vi "G heatmap=f(orbital angle, E_mol)_on Au.vi"() -> ()   [LabVIEW 2016]
uses:
  <vilib>/Math Plots/3D Math Plots/3D Contour/3D Contour XCtrl/3D Contour.xctl
  <vilib>/Math Plots/3D Math Plots/3D Contour/3D Contour Datatype/3D Contour Datatype.lvclass
  <vilib>/Analysis/1siggen.llb/Ramp Pattern by Samples.vi
  <vilib>/Math Plots/3D Math Plots/3D Contour/3D Contour Datatype/Public/Plot Helper (Vector).vi
  <vilib>/Utility/file.llb/Write Delimited Spreadsheet (DBL).vi
  <vilib>/Analysis/NI_AALBase.lvlib
  <vilib>/Math Plots/3D Math Plots/3D Plot/3D Plot Datatype/3D Plot Datatype.lvclass
  <vilib>/Analysis/NI_AALPro.lvlib
panel:
  out "SDOS(angle, e_iso) for t(d-head)_sum dz2 & dyz 2":refnum<class "3D Plot Datatype.lvclass">[](xcontrol)
  out "unweighted pz SDOS \n@ intercept":dbl
  out "t^2_pz-mol":dbl
  out "t_pz-mol":dbl
  in  "eta (pp sigma)":i32=2
  in  "t_pz band":dbl=4.15 format="%.2f"
  in  "e_pz band (vs. E_F)":dbl=8.19 format="%.2f"
  out "pz SDOS top (/eV/atom)":dbl=0.118 format="%.3f"
  in  "turn on dyz":bool=TRUE
  in  "turn on dz2":bool=TRUE
  out "<= min[dnn]?":bool
  out "e_FMO after dz2\n(vs. E_F) <=>\nintercept on E\ndz2 band-mol":dbl
  out "e_FMO after sp \n(vs. E_F) <=>\nintercept on E\nsp band-mol":dbl
  out "intercept on E\ndyz band-mol":dbl
  out "graphical sol_dyz band-mol":cluster{"Ramp Pattern":dbl[], dbl[]}[](graph)
  out "delta shift by d band \n(w.r.t. e_FMO coupled to s/p then dz2 )":dbl
  out "unweighted dyz SDOS \n@intercept":dbl
  in  "e_dyz band \n(vs. E_F)":dbl=-3.41 format="%.2f"
  in  "t_dyz band":dbl=1.1 format="%.2f"
  out "dyz SDOS top \n(/eV/atom)":dbl=0.793 format="%.3f"
  out "log(G/G0)=f(angle, e_iso) for t(sp-head)":refnum<class "3D Plot Datatype.lvclass">[](xcontrol)
  in  "min dnn (A)\nby induction":dbl=2.1 format="%.3g"
  out "peak value":dbl
  out "unweighted pxy SDOS \n@ intercept":dbl
  out "t^2_pxy-mol":dbl
  out "pxy SDOS top (/eV/atom)":dbl=0.118 format="%.3f"
  in  "e_pxy band (vs. E_F)":dbl=11.01 format="%.2f"
  in  "t_pxy band":dbl=6.11 format="%.2f"
  out "angle > ini?":bool
  in  "dnn shrinking \nrate\n(A/increment)":dbl=0.0094 format="%.4g"
  in  "induction rate\n(_-fold of increment)":dbl=1.9850000000000005 format="%.3g"
  in  "orbital angle \nstarting induction":dbl=46.809999999999995 format="%.2g"
  out "unweighted dz2 SDOS \n@intercept":dbl
  out "unweighted s SDOS \n@ intercept":dbl
  out "dz2 SDOS top \n(/eV/atom)":dbl=0.793 format="%.3f"
  out "s SDOS top (/eV/atom)":dbl=0.118 format="%.3f"
  in  "eta scaling for sp":dbl=0.417 format="%.3f"
  in  "name (d band)":string="on Au 5dz2 5dyz"
  in  "saving path_heatmap (d band)":path=path "C:/Users/NTU/Desktop/project_BiUPD & PbUPD/modelling/general heatmap all head_on Au"
  in  "save heatmap \n(d band)?":bool
  out "final ELA(angle, e_iso  for t(sp-head))":refnum<class "3D Plot Datatype.lvclass">[](xcontrol)
  out "delta(angle, e_iso) for t(d-head)_sum dz2 & dyz":refnum<class "3D Plot Datatype.lvclass">[](xcontrol)
  out "delta(angle, e_iso) for t(sp-head)_only s":refnum<class "3D Plot Datatype.lvclass">[](xcontrol)
  out "delta shift by dz2 band \n(w.r.t. e_FMO coupled to s/p )":dbl
  out "delta shift by sp band":dbl
  in  "dnn (pi) dyz":dbl=2.57 format="%0.2f"
  out "Gamma(angle, e_iso) for t(sp-head)_sum s pz py":refnum<class "3D Plot Datatype.lvclass">[](xcontrol)
  out "e_FMO \n(vs. E_F)":dbl
  out "log(G/G0) matrix":dbl[][](array[numeric])
  in  "tilt (mol axis - Z axis)":dbl format="%0.2f"
  out "final ELA(angle, e_iso)  for t(d-head)":refnum<class "3D Plot Datatype.lvclass">[](xcontrol)
  out "Gamma(angle, e_iso) for t(d-head)_sum dz2 & dyz":refnum<class "3D Plot Datatype.lvclass">[](xcontrol)
  out "log(G/G0)=f(angle, e_iso) for t(d-head)":refnum<class "3D Plot Datatype.lvclass">[](xcontrol)
  out "e_FMO (y)":dbl[](array[numeric])
  out "angle\narray\nfor sigma":dbl[](array[numeric])
  in  "create heatmap":bool=TRUE
  in  "name (sp band)":string="on Au 6s 6pxy"
  in  "save heatmap \n(sp band)?":bool
  in  "saving path_heatmap (sp band)":path=path "C:/Users/NTU/Desktop/project_BiUPD & PbUPD/modelling/general heatmap all head_on Au"
  in  "lower angle":dbl=-90.0 format="%_3g"
  in  "upper angle":dbl=90.0 format="%_3g"
  in  "angle increment":dbl=0.5 format="%_3g"
  in  "lower e_iso FMO":dbl=-3.0 format="%_3g"
  in  "upper e_iso FMO":dbl=3.0 format="%_3g"
  in  "increment_iso FMO":dbl=0.03 format="%_3g"
  out "t^2_dz2-mol":dbl
  out "FWHM (eV)":dbl
  in  "dnn (pi)":dbl=2.57 format="%0.2f"
  in  "WF (eV) vs. Fermi":dbl format="%.2f"
  out "t^2_p-mol":dbl
  out "t_pxy-mol":dbl
  in  "eta (pp pi)":i32=3
  in  "start (eV)":dbl=-20.0 format="%.2f"
  in  "dnn (sigma)":dbl=2.57 format="%0.2f"
  in  "eta (sp sigma)":i32=1
  out "t_s-mol":dbl
  out "intercept on E\nsp band-mol":dbl
  out "graphical sol_sp band-mol":cluster{"Ramp Pattern":dbl[], dbl[]}[](graph)
  in  "e_s band (vs. E_F)":dbl=-0.04 format="%.2f"
  in  "t_s band":dbl=5.03 format="%.2f"
  out "E":dbl[](array[numeric])
  out "t^2_dyz-mol":dbl
  out "final ELA (eV), via \n(1) sp intercept\n(2) dz2 intercept\n(3) dyz intercept":dbl
  in  "ELD AO (pi w/ FMO) - Z axis":dbl format="%0.2f"
  out "graphical sol_dz2 band-mol":cluster{"Ramp Pattern":dbl[], dbl[]}[](graph)
  out "intercept on E\ndz2 band-mol":dbl
  out "t_dz2-mol":dbl
  out "t_dyz-mol":dbl
  in  "e_dz2 band \n(vs. E_F)":dbl=-3.8000000000000003 format="%.2f"
  in  "t_dz2 band":dbl=1.26 format="%.2f"
  in  "eta (pi)":i32=2
  in  "ELD AO (sigma w/ FMO) - Z axis":dbl format="%0.2f"
  in  "mol backbone (# n)":dbl=8.0 format="%.2f"
  in  "beta (per n)":dbl=1.0 format="%.2f"
  out "conductance G0 \n(on E_F, low bias)":dbl format="%#.3e"
  in  "eta (sigma)":i32=1
  out "transmission T(E)":cluster{"Ramp Pattern":dbl[], dbl[]}(graph)
  in  "d state R (Ang)":dbl=1.0099999999999998 format="%0.2f"
  in  "FMO - mol axis":dbl format="%0.2f"
  in  "dnn (sigma) dz2":dbl=2.57 format="%0.2f"
  in  "samples":i32=10000
  in  "end (eV)":dbl=20.0 format="%_3g"
  # "for eld-head hopping integral: \nHarrsion and S-K"
  # "for ELA & Gamma: Hilbert & Newns-Anderson-Grimley graphical method"
  # "for T(E) and G(E_F)\nLandauer formula"
  # "logG heatmap = f(t(number basis), e_iso FMO)"
  # "step2. dz2 band-mol \ncoupling"
  # "step1. s/p band-mol coupling"
  # "step3. dyz band-mol coupling"
  # "Harrison LCAO hopping integral (V)"
  # "exp decay for backbone"
  # "internuclear \nspacing, dnn (Ang)"
  # "off-diagonal element type"
  # "Au s\nc: -0.04\nt: 5.03"
  # "1 sp_sigma\n2 pp_sigma"
  # "FMO-s/p eld AO"
  # "1 sp_sigma\n2 pp_sigma"
  # "Au pz\nc: 8.19\nt: 4.15"
  # "1 sp_pi =0\n2 pp_sigma\n3 pp_pi"
  # "FMO-d eld AO"
  # "Au py\nc: 11.01\nt: 6.11"
  # "1 pd_sigma\n2 pd_pi"
  # "Au dz2\nc: -3.80\nt: 1.26"
  # "Au dyz\nc: -3.41\nt: 1.10"
  # "the avg of the two \nshould be e_ELD (vs. E_F)"
  # "1 pd_sigma\n2 pd_pi"
  # "to switch off certain interactions => set very large d (Ang)"
  # "for heatmap"
  # "for inducting effect"
  # "e_iso FMO\n (vs. E_F)"
  # "angle basis"
  # "induction"
  # "dnn"
  # "note: this is\nnot simply \nthe Gamma"
  # "to switch off certain effects => set 1 or 0"
  # "Slater-Koster t =f(bond angle)"
  # "+"
  # "一"
  # "FMO - ELD AO \nangle (sigma)"
  # "="
  # "FMO - ELD AO\n angle (pi)"
  # "="
  # "inverse \ncolor scale"
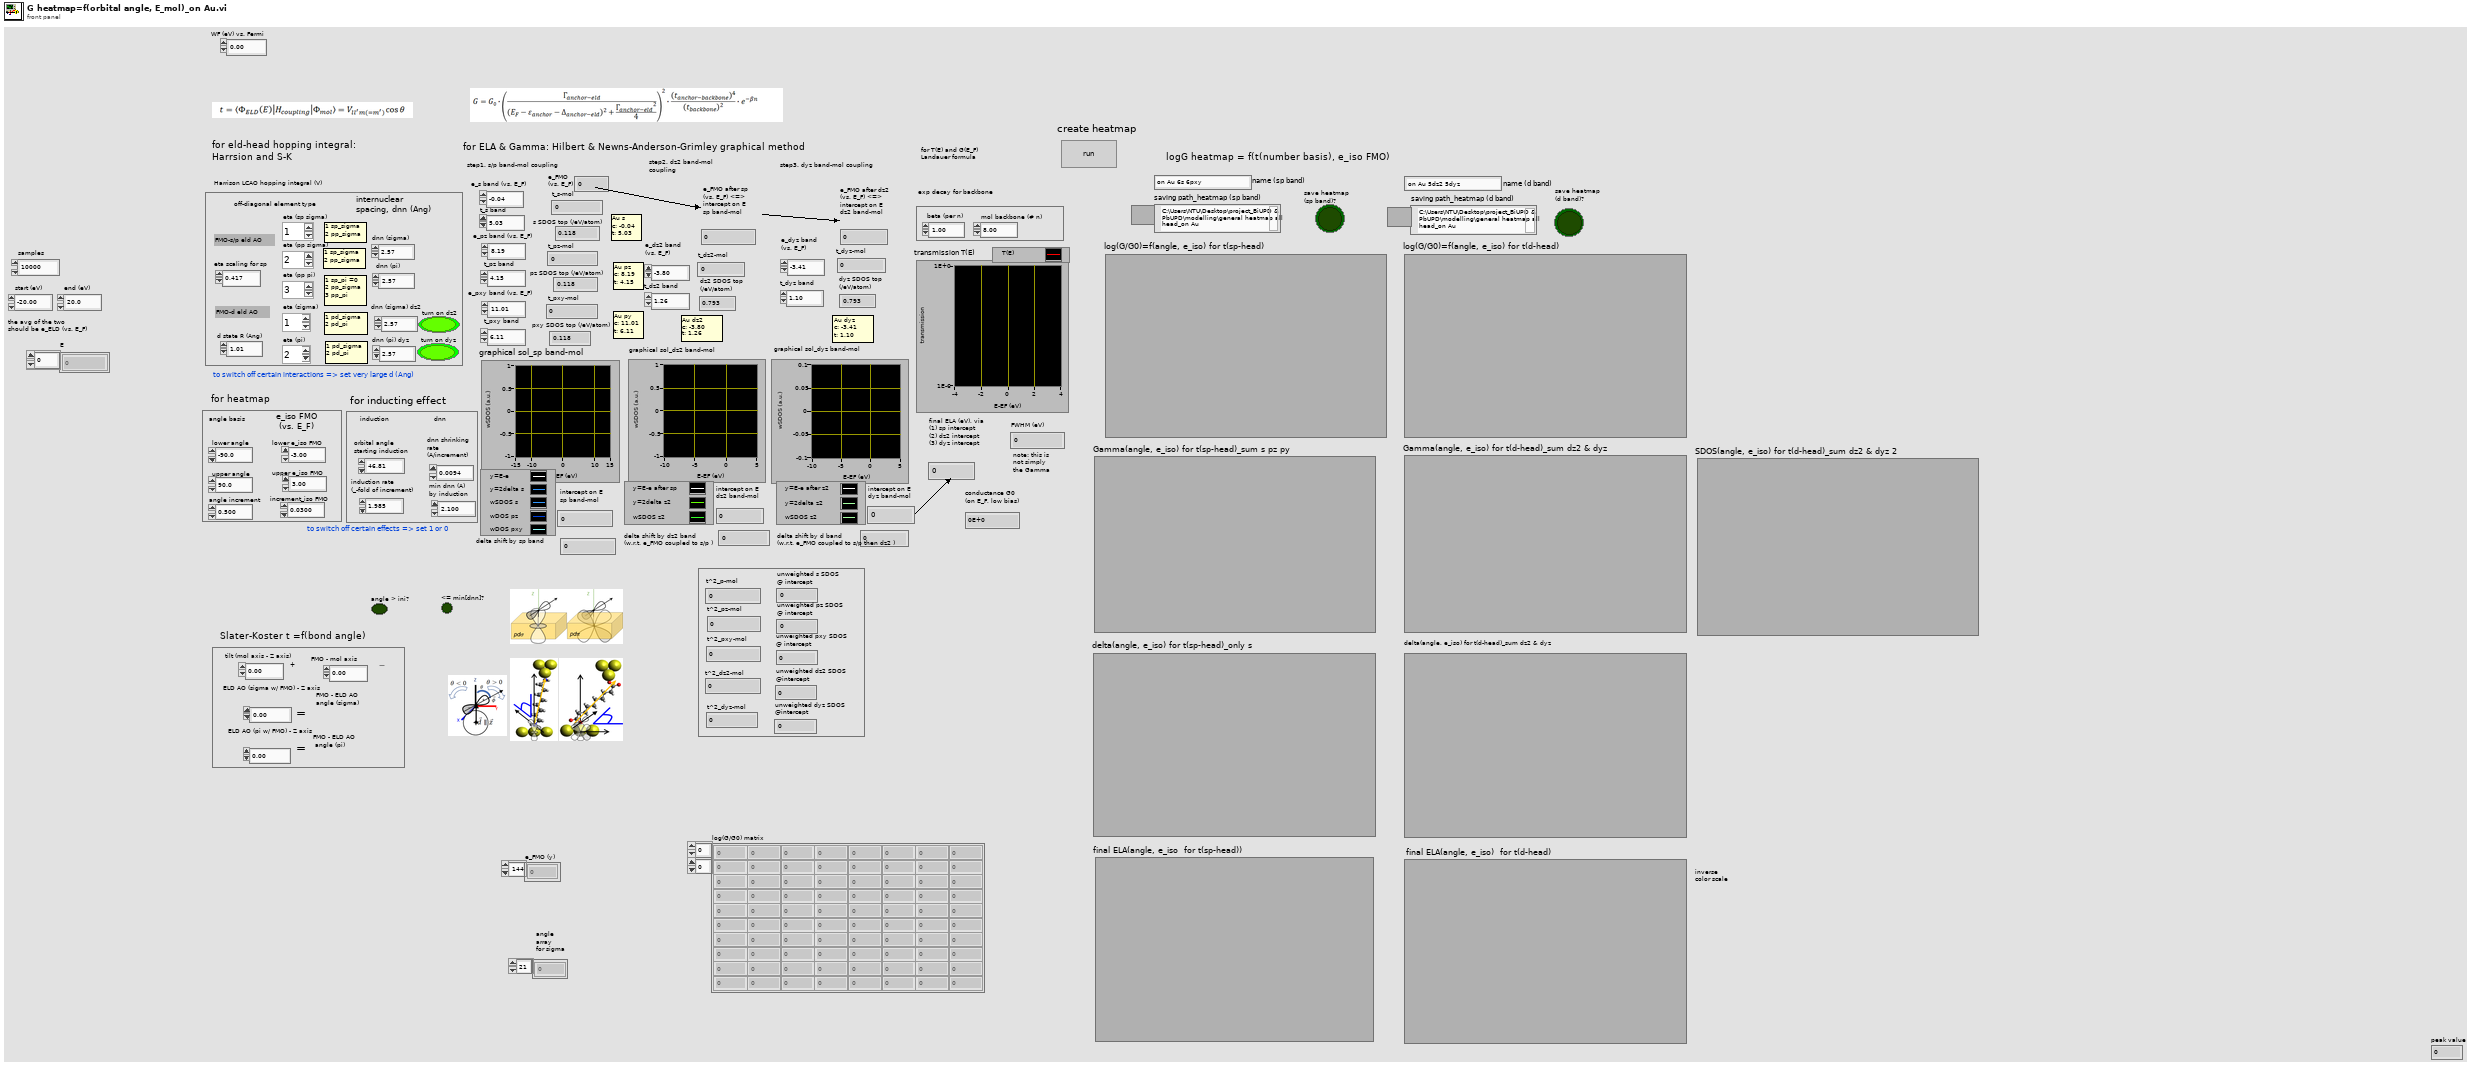
[diagram p1: front panel]
types:
  T1 = cluster{"Ramp Pattern":dbl[], "Hilbert{X}":dbl[]}
  T2 = cluster{"Ramp Pattern":dbl[], "Hilbert{X}":dbl[]}[]
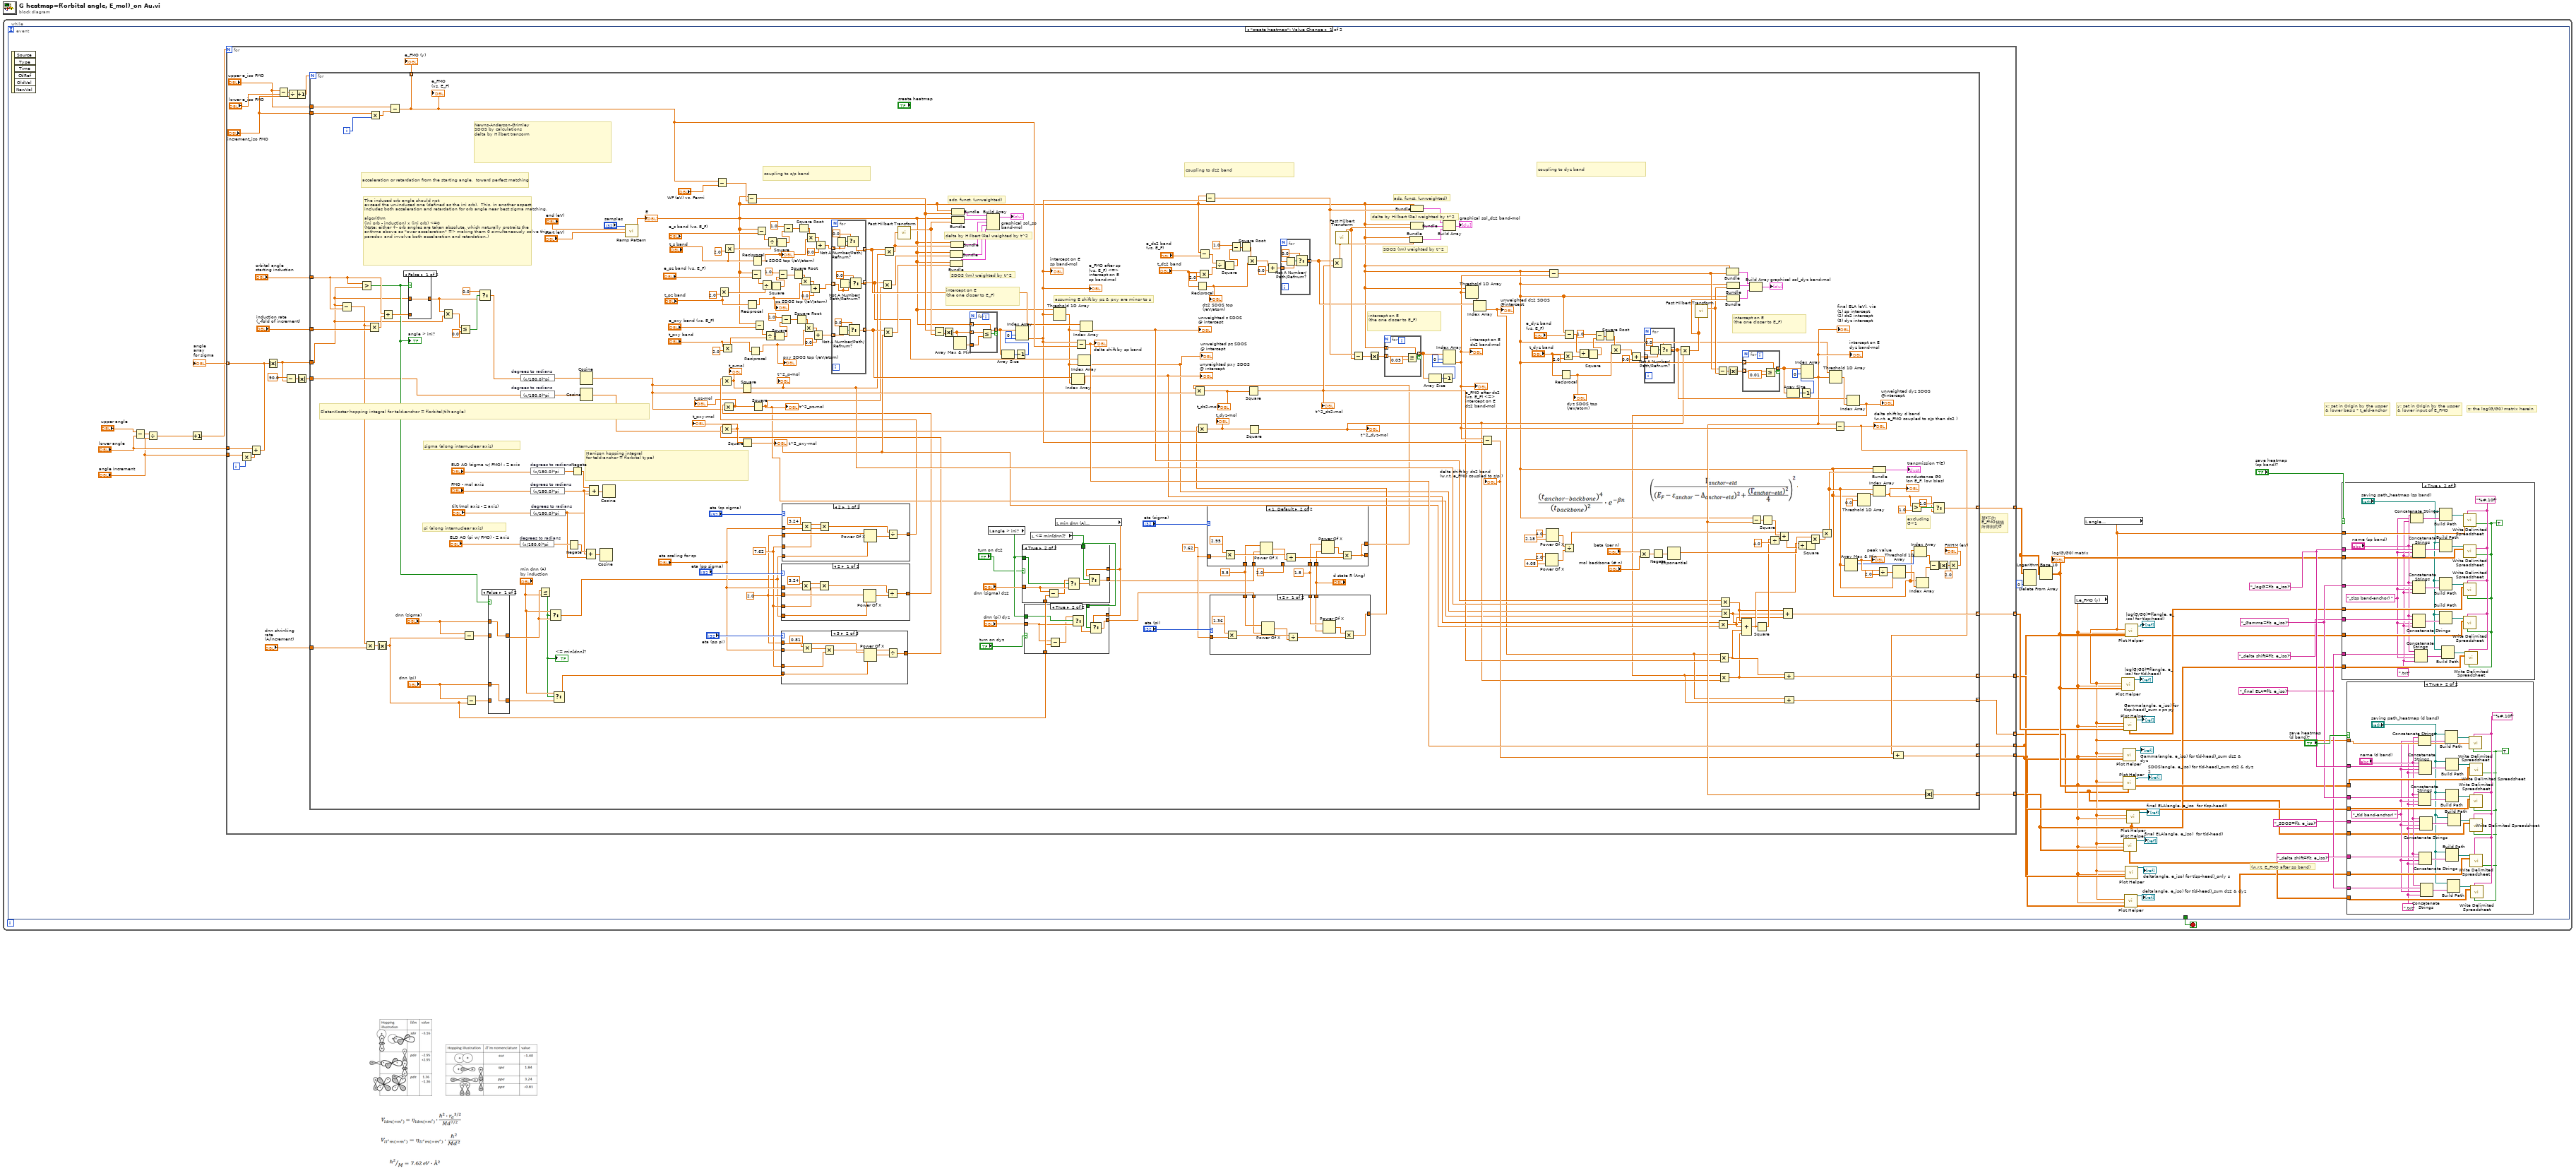
[diagram p0: block diagram]
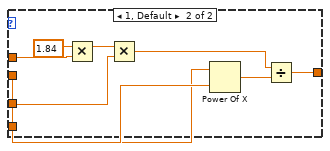
[diagram p4: hidden frame]
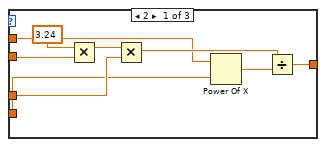
[diagram p9: hidden frame]
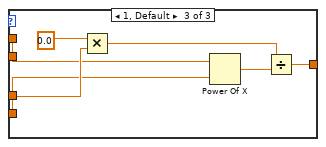
[diagram p10: hidden frame]
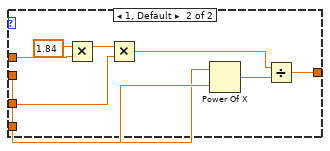
[diagram p11: hidden frame]
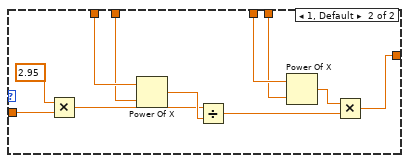
[diagram p12: hidden frame]
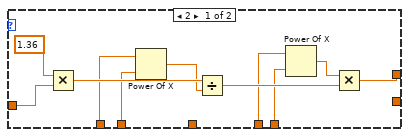
[diagram p13: hidden frame]
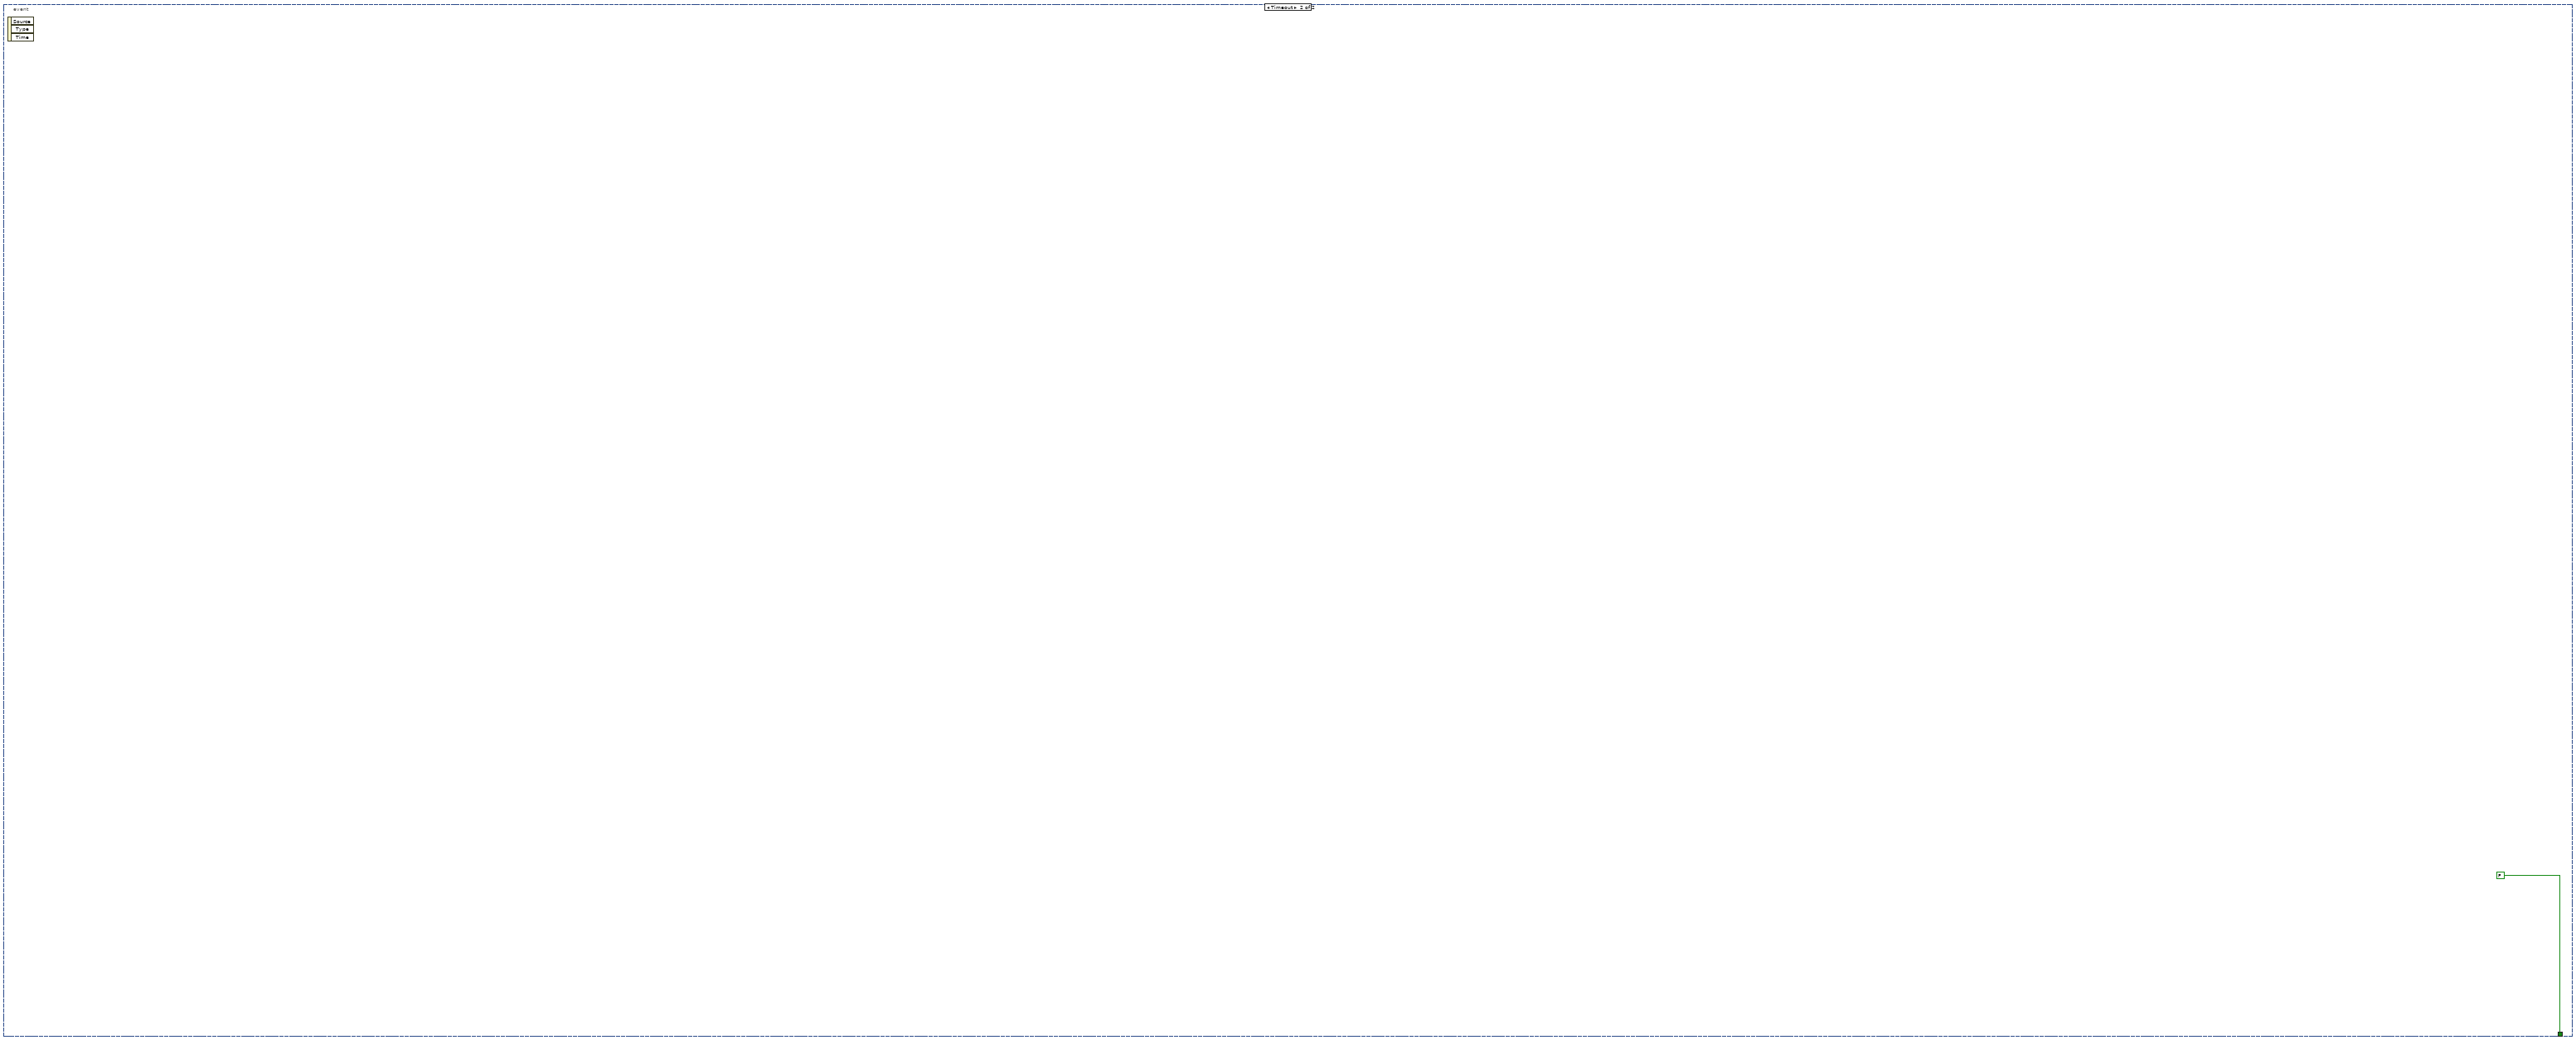
[diagram p14: hidden frame]
diagram:
  n1 = while {
    stop <- w1 stop-if-true
    n2 = event shown="[0] \"create heatmap\": Value Change" {
      selector: _ -> [_ _]
      dyn-events: _ -> [_ _]
      timeout: _ -> [_ _]
      tunnel: [_ FALSE] -> w1
      event "create heatmap": Value Change {
        w20 = "_logG=f(t, e_iso)" ("string")
        w16 = "_final ELA=f(t, e_iso)" ("string")
        w19 = "_Gamma=f(t, e_iso)" ("string")
        # "(w.r.t. E_FMO after sp band)"
        # "z: the log(G/G0) matrix herein"
        # "y: set in Origin by the upper \n& lower input of E_FMO"
        # "x: set in Origin by the upper\n& lower basis * t_eld-anchor"
        n3 = event-data() -> ()  [unwired: 1 in, 6 out]
        n4 = Subtract(x="upper angle", y="lower angle") -> (x-y=w35:dbl)
        n5 = Divide(x=w35, y="angle increment") -> (x/y=w36:dbl)
        n6 = Increment(x=w36) -> (x+1=w28:dbl)
        n7 = for {
          N: w28 -> [_]
          tunnel: "lower angle" -> [w106]
          tunnel: "angle increment" -> [w111]
          tunnel: [w101] -> w7 mode=indexing
          tunnel: [w96] -> w32 mode=indexing
          tunnel: [w109] -> w13 mode=indexing
          tunnel: [w108] -> w12 mode=indexing
          tunnel: [w104] -> w14 mode=indexing
          tunnel: [w103] -> w11 mode=indexing
          tunnel: [w102] -> w10 mode=indexing
          tunnel: [w91] -> w3 mode=indexing
          i -> [w112]
          # "某t下的\nE_FMO掃描\n所得到的G"
          n8 = Multiply(x=w111, y=w112) -> (x*y=w105:dbl)
          n9 = Add(x=w106, y=w105) -> (x+y=w96:dbl)
          n10 = Absolute Value(x=w96) -> (abs(x)=w94:dbl)
          n11 = Subtract(x="upper e_iso FMO", y="lower e_iso FMO") -> (x-y=w115:dbl)
          n12 = Subtract(x=90.0 ("y"), y=w94) -> (x-y=w95:dbl)
          n13 = Divide(x=w115, y="increment_iso FMO") -> (x/y=w116:dbl)
          n14 = Increment(x=w116) -> (x+1=w107:dbl)
          n15 = Absolute Value(x=w95) -> (abs(x)=w93:dbl)
          n16 = for {
            N: w107 -> [_]
            tunnel: "upper e_iso FMO" -> [w338]
            tunnel: "increment_iso FMO" -> [w337]
            tunnel: [w328] -> w110 mode=indexing
            tunnel: [w176] -> w109 mode=indexing
            tunnel: [w313] -> w108 mode=indexing
            tunnel: w94 -> [w225]
            tunnel: [w179] -> w104 mode=indexing
            tunnel: [w329] -> w103 mode=indexing
            tunnel: [w173] -> w102 mode=indexing
            tunnel: [w231] -> w101 mode=indexing
            tunnel: "orbital angle \nstarting induction" -> [w273]
            tunnel: "induction rate\n(_-fold of increment)" -> [w272]
            tunnel: "dnn shrinking \nrate\n(A/increment)" -> [w270]
            tunnel: w93 -> [w216]
            tunnel: [w117] -> w91 mode=indexing
            i -> [w339]
            w136 = 7.62
            w135 = 2.0
            w358 = 1.5
            w360 = 3.5
            w359 = 7.62
            # "acceleration or retardation from the starting angle,  toward perfect matching"
            # "intercept on E \n(the one closer to E_F)"
            # "coupling to dyz band"
            # "The induced orb angle should not \nexceed the un-induced one (defined as the ini orb).  This, in another aspect, includes both acceleration and retardation for orb angle near best sigma matching.\n\nalgorithm\n(ini orb - induction) x (ini orb) <=0\n(Note: either +- orb angles are taken absolute, which naturally protraits the arithma above as \"over acceleration\" => making them 0 simultaneously solve this paradox and involve both acceleration and retardation.)"
            # "assuming E shift by pz & pxy are minor to s"
            # "excluding\nG>1"
            # "SDOS (Im) weighted by t^2"
            # "delta by Hilbert (Re) weighted by t^2"
            # "ads. funct. (unweighted)"
            # "SDOS (Im) weighted by t^2"
            # "delta by Hilbert (Re) weighted by t^2"
            # "ads. funct. (unweighted)"
            # "Newns-Anderson-Grimley \nSDOS by calculations\ndelta by Hilbert transorm"
            # "intercept on E \n(the one closer to E_F)"
            # "intercept on E \n(the one closer to E_F)"
            # "coupling to dz2 band"
            # "coupling to s/p band"
            # "Harrison hopping integral \nfor teld-anchor = f(orbital type)"
            # "pi (along internuclear axis)"
            # "sigma (along internuclear axis)"
            # "Slater-Koster hopping integral for teld-anchor = f(orbital/tilt angle)"
            n17 = Subtract(x=w225, y=w273) -> (x-y=w157:dbl)
            n18 = Greater?(x=w273, y=w225) -> (0:w267:bool)
            "angle > ini?" <- w267
            n19 = Multiply(x=w157, y=w270) -> (x*y=w271:dbl)
            n20 = Multiply(x=w157, y=w272) -> (x*y=w275:dbl)
            n21 = Multiply(x=w337, y=w339) -> (x*y=w340:dbl)
            n22 = Absolute Value(x=w271) -> (abs(x)=w264:dbl)
            n23 = Add(x=w273, y=w275) -> (x+y=w274:dbl)
            n24 = Subtract(x=w338, y=w340) -> (x-y=w328:dbl)
            "e_FMO \n(vs. E_F)" <- w328
            n25 = case shown="False" w267 {
              tunnel: w225 -> [w441 _]
              tunnel: [w441 w442] -> w226
              tunnel: w274 -> [_ w442]
              frame False {
              }
              frame True {
              }
            }
            n26 = Multiply(x=w226, y=w225) -> (x*y=w229:dbl)
            n27 = Less Or Equal?(x=w229, y=0.0) -> (x <= y?=w227:bool)
            n28 = Subtract(x="dnn (sigma)", y=w264) -> (x-y=w269:dbl)
            n29 = Subtract(x="dnn (pi)", y=w264) -> (x-y=w268:dbl)
            n30 = Select(t=0.0 ("y"), s=w227, f=w226) -> (s? t:f=w219:dbl)
            n31 = case shown="False" w267 {
              tunnel: w269 -> [_ w440]
              tunnel: [w438 w440] -> w224
              tunnel: w268 -> [_ w439]
              tunnel: [w437 w439] -> w223
              tunnel: "dnn (sigma)" -> [w438 _]
              tunnel: "dnn (pi)" -> [w437 _]
              frame False {
              }
              frame True {
              }
            }
            n32 = expression code="(x/180.0)*pi" "degrees to radians"("ELD AO (pi w/ FMO) - Z axis") -> (w375:dbl)
            n33 = expression code="(x/180.0)*pi" "degrees to radians"(w219) -> (w277:dbl)
            n34 = expression code="(x/180.0)*pi" "degrees to radians"(w216) -> (w276:dbl)
            n35 = expression code="(x/180.0)*pi" "degrees to radians"("ELD AO (sigma w/ FMO) - Z axis") -> (w379:dbl)
            n36 = expression code="(x/180.0)*pi" "degrees to radians"("FMO - mol axis") -> (w373:dbl)
            n37 = expression code="(x/180.0)*pi" "degrees to radians"("tilt (mol axis - Z axis)") -> (w341:dbl)
            n38 = Less Or Equal?(x=w224, y="min dnn (A)\nby induction") -> (x <= y?=w221:bool)
            "<= min[dnn]?" <- w221
            n39 = Select(t="min dnn (A)\nby induction", s=w221, f=w224) -> (s? t:f=w134:dbl)
            n40 = Select(t="min dnn (A)\nby induction", s=w221, f=w223) -> (s? t:f=w220:dbl)
            n41 = Negate(x=w375) -> (-x=w374:dbl)
            n42 = Negate(x=w379) -> (-x=w376:dbl)
            n43 = Cosine(x=w277) -> (cos(x)=w128:dbl)
            n44 = Cosine(x=w276) -> (cos(x)=w278:dbl)
            n45 = Compound Arithmetic op=ADD(w374, w373, w341) -> (w377:dbl)
            n46 = Compound Arithmetic op=ADD(w376, w373, w341) -> (w382:dbl)
            n47 = Cosine(x=w377) -> ()  [unwired: 1 out]
            n48 = Cosine(x=w382) -> ()  [unwired: 1 out]
            n49 = call-poly <vilib>:"Ramp Pattern.vi"("start"="start (eV)", "end"="end (eV)", "samples"="samples") -> ("Ramp Pattern"=w142:dbl[])  [unwired: 7 in, 1 out]
            "E" <- w142
            n50 = Subtract(x=w328, y="WF (eV) vs. Fermi") -> (x-y=w342:dbl)
            n51 = Multiply(x="t_pz band", y=2.0) -> (x*y=w154:dbl)
            n52 = Multiply(x="t_pxy band", y=2.0) -> (x*y=w261:dbl)
            n53 = Multiply(x="t_s band", y=2.0) -> (x*y=w263:dbl)
            n54 = Subtract(x=w142, y=w342) -> (x-y=w383:dbl[])
            n55 = Reciprocal(x="t_pz band") -> (1/x=w155:dbl)
            "pz SDOS top (/eV/atom)" <- w155
            n56 = Reciprocal(x="t_pxy band") -> (1/x=w251:dbl)
            "pxy SDOS top (/eV/atom)" <- w251
            n57 = Subtract(x=w142, y="e_pz band (vs. E_F)") -> (x-y=w145:dbl[])
            n58 = Reciprocal(x="t_s band") -> (1/x=w262:dbl)
            "s SDOS top (/eV/atom)" <- w262
            n59 = Subtract(x=w142, y="e_pxy band (vs. E_F)") -> (x-y=w253:dbl[])
            n60 = Subtract(x=w142, y="e_s band (vs. E_F)") -> (x-y=w311:dbl[])
            n61 = Divide(x=w145, y=w154) -> (x/y=w147:dbl[])
            n62 = Divide(x=w253, y=w261) -> (x/y=w255:dbl[])
            n63 = Divide(x=w311, y=w263) -> (x/y=w309:dbl[])
            n64 = Square(x=w147) -> (x^2=w148:dbl[])
            n65 = Square(x=w255) -> (x^2=w256:dbl[])
            n66 = Square(x=w309) -> (x^2=w308:dbl[])
            n67 = Subtract(x=1.0, y=w148) -> (x-y=w149:dbl[])
            n68 = Subtract(x=1.0, y=w256) -> (x-y=w257:dbl[])
            n69 = case shown="3" "eta (pp pi)" {
              tunnel: w136 -> [w463 w473 w480]
              tunnel: [w462 w472 w479] -> w132
              tunnel: w135 -> [w464 w471 w478]
              tunnel: w220 -> [w461 w470 w477]
              tunnel: "eta scaling for sp" -> [w459 w468 _]
              frame 2 {
                n70 = Multiply(x=3.24, y=w459) -> (x*y=w460:dbl)
                n71 = Multiply(x=w460, y=w463) -> (x*y=w466:dbl)
                n72 = Power Of X(1:w461, 2:w464) -> (0:w465:dbl)
                n73 = Divide(x=w466, y=w465) -> (x/y=w462:dbl)
              }
              frame 3 {
                n74 = Multiply(x=0.81, y=w468) -> (x*y=w469:dbl)
                n75 = Multiply(x=w469, y=w473) -> (x*y=w475:dbl)
                n76 = Power Of X(1:w470, 2:w471) -> (0:w476:dbl)
                n77 = Divide(x=w475, y=w476) -> (x/y=w472:dbl)
              }
              frame 1, Default {
                n78 = Multiply(x=0.0, y=w480) -> (x*y=w482:dbl)
                n79 = Power Of X(1:w477, 2:w478) -> (0:w483:dbl)
                n80 = Divide(x=w482, y=w483) -> (x/y=w479:dbl)
              }
            }
            n81 = Multiply(x=w132, y=w278) -> (x*y=w333:dbl)
            "t_pxy-mol" <- w333
            n82 = Square(x=w333) -> (x^2=w169:dbl)
            "t^2_pxy-mol" <- w169
            n83 = case shown="2" "eta (pp sigma)" {
              tunnel: w136 -> [w398 w409]
              tunnel: [w395 w406] -> w129
              tunnel: w134 -> [w396 w408]
              tunnel: w135 -> [w399 w407]
              tunnel: "eta scaling for sp" -> [w393 w402]
              frame 2 {
                n84 = Multiply(x=3.24, y=w393) -> (x*y=w394:dbl)
                n85 = Multiply(x=w394, y=w398) -> (x*y=w400:dbl)
                n86 = Power Of X(1:w396, 2:w399) -> (0:w401:dbl)
                n87 = Divide(x=w400, y=w401) -> (x/y=w395:dbl)
              }
              frame 1, Default {
                n88 = Multiply(x=1.84, y=w402) -> (x*y=w403:dbl)
                n89 = Multiply(x=w403, y=w409) -> (x*y=w405:dbl)
                n90 = Power Of X(1:w408, 2:w407) -> (0:w404:dbl)
                n91 = Divide(x=w405, y=w404) -> (x/y=w406:dbl)
              }
            }
            n92 = Multiply(x=w129, y=w128) -> (x*y=w127:dbl)
            "t_pz-mol" <- w127
            n93 = Square(x=w127) -> (x^2=w121:dbl)
            "t^2_pz-mol" <- w121
            n94 = Subtract(x=1.0, y=w308) -> (x-y=w307:dbl[])
            n95 = case shown="2" "eta (sp sigma)" {
              tunnel: w136 -> [w489 w500]
              tunnel: [w486 w497] -> w133
              tunnel: w134 -> [w487 w499]
              tunnel: w135 -> [w490 w498]
              tunnel: "eta scaling for sp" -> [w484 w493]
              frame 2 {
                n96 = Multiply(x=3.24, y=w484) -> (x*y=w485:dbl)
                n97 = Multiply(x=w485, y=w489) -> (x*y=w491:dbl)
                n98 = Power Of X(1:w487, 2:w490) -> (0:w492:dbl)
                n99 = Divide(x=w491, y=w492) -> (x/y=w486:dbl)
              }
              frame 1, Default {
                n100 = Multiply(x=1.84, y=w493) -> (x*y=w494:dbl)
                n101 = Multiply(x=w494, y=w500) -> (x*y=w496:dbl)
                n102 = Power Of X(1:w499, 2:w498) -> (0:w495:dbl)
                n103 = Divide(x=w496, y=w495) -> (x/y=w497:dbl)
              }
            }
            n104 = Multiply(x=w133, y=w128) -> (x*y=w332:dbl)
            "t_s-mol" <- w332
            n105 = Square(x=w332) -> (x^2=w171:dbl)
            "t^2_p-mol" <- w171
            n106 = Square Root(x=w149) -> (sqrt(x)=w150:dbl[])
            n107 = Square Root(x=w257) -> (sqrt(x)=w258:dbl[])
            n108 = Square Root(x=w307) -> (sqrt(x)=w306:dbl[])
            n109 = Multiply(x=w150, y=w155) -> (x*y=w151:dbl[])
            n110 = Multiply(x=w258, y=w251) -> (x*y=w259:dbl[])
            n111 = Multiply(x=w306, y=w262) -> (x*y=w305:dbl[])
            n112 = Add(x=w151, y=0.0) -> (x+y=w143:dbl[])
            n113 = Add(x=w259, y=0.0) -> (x+y=w249:dbl[])
            n114 = Add(x=w305, y=0.0) -> (x+y=w303:dbl[])
            n115 = for {
              tunnel: w303 -> [w455] mode=indexing
              tunnel: [w457] -> w217 mode=indexing
              tunnel: w249 -> [w452] mode=indexing
              tunnel: [w451] -> w218 mode=indexing
              tunnel: w143 -> [w448] mode=indexing
              tunnel: [w447] -> w126 mode=indexing
              n116 = Not A Number/Path/Refnum?(number/path/refnum=w455) -> (NaN/Path/Refnum?=w458:bool)
              n117 = Not A Number/Path/Refnum?(number/path/refnum=w452) -> (NaN/Path/Refnum?=w453:bool)
              n118 = Not A Number/Path/Refnum?(number/path/refnum=w448) -> (NaN/Path/Refnum?=w449:bool)
              n119 = Select(t=0.0, s=w458, f=w455) -> (s? t:f=w457:dbl)
              n120 = Select(t=0.0, s=w453, f=w452) -> (s? t:f=w451:dbl)
              n121 = Select(t=0.0, s=w449, f=w448) -> (s? t:f=w447:dbl)
            }
            n122 = Multiply(x=w126, y=w121) -> (x*y=w140:dbl[])
            n123 = Multiply(x=w218, y=w169) -> (x*y=w141:dbl[])
            n124 = Multiply(x=w217, y=w171) -> (x*y=w297:dbl[])
            n125 = call <vilib>:"Fast Hilbert Transform.vi"("X"=w297) -> ("Hilbert{X}"=w300:dbl[])  [unwired: 1 out]
            n126 = Subtract(x=w383, y=w300) -> (x-y=w352:dbl[])
            n127 = Absolute Value(x=w352) -> (abs(x)=w299:dbl[])
            n128 = Bundle("Ramp Pattern"=w142, w141) -> (w139:cluster{"Ramp Pattern":dbl[], dbl[]})  [unwired: 1 in]
            n129 = Bundle("Ramp Pattern"=w142, w140) -> (w234:cluster{"Ramp Pattern":dbl[], dbl[]})  [unwired: 1 in]
            n130 = Bundle("Ramp Pattern"=w142, w297) -> (w301:cluster{"Ramp Pattern":dbl[], dbl[]})  [unwired: 1 in]
            n131 = Bundle("Ramp Pattern"=w142, "Hilbert{X}"=w300) -> (w353:T1)  [unwired: 1 in]
            n132 = Bundle("Ramp Pattern"=w142, w383) -> (w355:cluster{"Ramp Pattern":dbl[], dbl[]})  [unwired: 1 in]
            n133 = Array Max & Min(array=w299) -> (min value=w298:dbl)  [unwired: 3 out]
            n134 = for {
              tunnel: w299 -> [w505] mode=indexing
              tunnel: [w503] -> w351 mode=indexing if=w504
              tunnel: w142 -> [w503] mode=indexing
              tunnel: w298 -> [w502]
              n135 = Less Or Equal?(x=w505, y=w502) -> (x <= y?=w504:bool)
            }
            n136 = Build Array(w355, w353, w301, w234, w139) -> (→"graphical sol_sp band-mol":T2)
            n137 = local read "angle > ini?"() -> (w165:bool)
            n138 = Array Size(array=w351) -> (size(s)=w349:i32)
            n139 = Decrement(x=w349) -> (x-1=w348:i32)
            n140 = Index Array(array=w351, index #1=0 ("index"), index #2=w348) -> (element #2=w182:dbl)  [unwired: 1 out]
            "intercept on E\nsp band-mol" <- w182
            "e_FMO after sp \n(vs. E_F) <=>\nintercept on E\nsp band-mol" <- w182
            n141 = local read "<= min[dnn]?"() -> (w161:bool)
            n142 = Threshold 1D Array(2:w182, 3:w142) -> (0:w125:dbl)  [unwired: 1 in]
            n143 = local read "min dnn (A)\nby induction"() -> (w160:dbl)
            n144 = case shown="True" "turn on dz2" {
              tunnel: w264 -> [_ w428]
              tunnel: "dnn (sigma) dz2" -> [w420 w427]
              tunnel: w165 -> [_ w425]
              tunnel: w161 -> [_ w424]
              tunnel: w160 -> [_ w423]
              tunnel: [w420 w421] -> w159
              frame False {
              }
              frame True {
                n145 = Subtract(x=w427, y=w428) -> (x-y=w426:dbl)
                n146 = Select(t=w426, s=w425, f=w427) -> (s? t:f=w422:dbl)
                n147 = Select(t=w423, s=w424, f=w422) -> (s? t:f=w421:dbl)
              }
            }
            n148 = case shown="True" "turn on dyz" {
              tunnel: w264 -> [_ w419]
              tunnel: w165 -> [_ w418]
              tunnel: "dnn (pi) dyz" -> [w411 w417]
              tunnel: [w411 w412] -> w158
              tunnel: w161 -> [_ w415]
              tunnel: w160 -> [_ w414]
              frame False {
              }
              frame True {
                n149 = Subtract(x=w417, y=w419) -> (x-y=w416:dbl)
                n150 = Select(t=w416, s=w418, f=w417) -> (s? t:f=w413:dbl)
                n151 = Select(t=w414, s=w415, f=w413) -> (s? t:f=w412:dbl)
              }
            }
            n152 = Index Array(array=w218, index=w125) -> (element=w170:dbl)
            "unweighted pxy SDOS \n@ intercept" <- w170
            n153 = Subtract(x=w182, y=w328) -> (x-y=w329:dbl)
            "delta shift by sp band" <- w329
            n154 = Index Array(array=w126, index=w125) -> (element=w122:dbl)
            "unweighted pz SDOS \n@ intercept" <- w122
            n155 = Index Array(array=w217, index=w125) -> (element=w172:dbl)
            "unweighted s SDOS \n@ intercept" <- w172
            n156 = Reciprocal(x="t_dz2 band") -> (1/x=w212:dbl)
            "dz2 SDOS top \n(/eV/atom)" <- w212
            n157 = Multiply(x="t_dz2 band", y=2.0) -> (x*y=w286:dbl)
            n158 = Subtract(x=w142, y="e_dz2 band \n(vs. E_F)") -> (x-y=w288:dbl[])
            n159 = Subtract(x=w142, y=w182) -> (x-y=w385:dbl[])
            n160 = case shown="1, Default" "eta (sigma)" {
              tunnel: w359 -> [w533 w549]
              tunnel: [w528 w539] -> w131
              tunnel: w159 -> [w531 w544]
              tunnel: w360 -> [w532 w543]
              tunnel: w358 -> [w530 w542]
              tunnel: "d state R (Ang)" -> [w529 w541]
              tunnel: 2.0 -> [_ _]
              tunnel: [_ w539] -> _
              frame 2 {
                n161 = Multiply(x=1.36, y=w533) -> (x*y=w535:dbl)
                n162 = Power Of X(1:w531, 2:w532) -> (0:w534:dbl)
                n163 = Divide(x=w535, y=w534) -> (x/y=w536:dbl)
                n164 = Power Of X(1:w529, 2:w530) -> (0:w537:dbl)
                n165 = Multiply(x=w537, y=w536) -> (x*y=w528:dbl)
              }
              frame 1, Default {
                n166 = Multiply(x=2.95, y=w549) -> (x*y=w547:dbl)
                n167 = Power Of X(1:w544, 2:w543) -> (0:w548:dbl)
                n168 = Divide(x=w547, y=w548) -> (x/y=w546:dbl)
                n169 = Power Of X(1:w541, 2:w542) -> (0:w545:dbl)
                n170 = Multiply(x=w545, y=w546) -> (x*y=w539:dbl)
              }
            }
            n171 = Multiply(x=w131, y=w128) -> (x*y=w335:dbl)
            "t_dz2-mol" <- w335
            n172 = case shown="2" "eta (pi)" {
              tunnel: w359 -> [w511 w527]
              tunnel: [w510 w522] -> w130
              tunnel: w360 -> [w509 w520]
              tunnel: w158 -> [w508 w519]
              tunnel: w358 -> [w507 w518]
              tunnel: "d state R (Ang)" -> [w506 w517]
              frame 2 {
                n173 = Multiply(x=1.36, y=w511) -> (x*y=w513:dbl)
                n174 = Power Of X(1:w508, 2:w509) -> (0:w512:dbl)
                n175 = Divide(x=w513, y=w512) -> (x/y=w514:dbl)
                n176 = Power Of X(1:w506, 2:w507) -> (0:w515:dbl)
                n177 = Multiply(x=w515, y=w514) -> (x*y=w510:dbl)
              }
              frame 1, Default {
                n178 = Multiply(x=2.95, y=w527) -> (x*y=w525:dbl)
                n179 = Power Of X(1:w519, 2:w520) -> (0:w526:dbl)
                n180 = Divide(x=w525, y=w526) -> (x/y=w524:dbl)
                n181 = Power Of X(1:w517, 2:w518) -> (0:w523:dbl)
                n182 = Multiply(x=w523, y=w524) -> (x*y=w522:dbl)
              }
            }
            n183 = Multiply(x=w130, y=w278) -> (x*y=w334:dbl)
            "t_dyz-mol" <- w334
            n184 = Divide(x=w288, y=w286) -> (x/y=w290:dbl[])
            n185 = Square(x=w290) -> (x^2=w291:dbl[])
            n186 = Subtract(x=1.0, y=w291) -> (x-y=w292:dbl[])
            n187 = Square Root(x=w292) -> (sqrt(x)=w293:dbl[])
            n188 = Multiply(x=w293, y=w212) -> (x*y=w294:dbl[])
            n189 = Square(x=w335) -> (x^2=w168:dbl)
            "t^2_dz2-mol" <- w168
            n190 = Square(x=w334) -> (x^2=w167:dbl)
            "t^2_dyz-mol" <- w167
            n191 = Add(x=w294, y=0.0) -> (x+y=w296:dbl[])
            n192 = for {
              tunnel: w296 -> [w443] mode=indexing
              tunnel: [w445] -> w215 mode=indexing
              n193 = Not A Number/Path/Refnum?(number/path/refnum=w443) -> (NaN/Path/Refnum?=w446:bool)
              n194 = Select(t=0.0, s=w446, f=w443) -> (s? t:f=w445:dbl)
            }
            n195 = Multiply(x=w215, y=w168) -> (x*y=w283:dbl[])
            n196 = call <vilib>:"Fast Hilbert Transform.vi"("X"=w283) -> ("Hilbert{X}"=w285:dbl[])  [unwired: 1 out]
            n197 = Subtract(x=w385, y=w285) -> (x-y=w368:dbl[])
            n198 = Absolute Value(x=w368) -> (abs(x)=w282:dbl[])
            n199 = for {
              tunnel: w282 -> [w553] mode=indexing
              tunnel: [w551] -> w367 mode=indexing if=w552
              tunnel: w142 -> [w551] mode=indexing
              n200 = Less Or Equal?(x=w553, y=0.05) -> (x <= y?=w552:bool)
            }
            n201 = Bundle("Ramp Pattern"=w142, w283) -> (w284:cluster{"Ramp Pattern":dbl[], dbl[]})  [unwired: 1 in]
            n202 = Bundle("Ramp Pattern"=w142, w385) -> (w371:cluster{"Ramp Pattern":dbl[], dbl[]})  [unwired: 1 in]
            n203 = Bundle("Ramp Pattern"=w142, "Hilbert{X}"=w285) -> (w369:T1)  [unwired: 1 in]
            n204 = Array Size(array=w367) -> (size(s)=w365:i32)
            n205 = Decrement(x=w365) -> (x-1=w364:i32)
            n206 = Index Array(array=w367, index #1=0 ("index"), index #2=w364) -> (element #2=w181:dbl)  [unwired: 1 out]
            "intercept on E\ndz2 band-mol" <- w181
            "e_FMO after dz2\n(vs. E_F) <=>\nintercept on E\ndz2 band-mol" <- w181
            n207 = Build Array(w371, w369, w284) -> (→"graphical sol_dz2 band-mol":T2)
            n208 = Threshold 1D Array(2:w181, 3:w142) -> (0:w214:dbl)  [unwired: 1 in]
            n209 = Index Array(array=w215, index=w214) -> (element=w119:dbl)
            "unweighted dz2 SDOS \n@intercept" <- w119
            n210 = Subtract(x=w181, y=w182) -> (x-y=w175:dbl)
            "delta shift by dz2 band \n(w.r.t. e_FMO coupled to s/p )" <- w175
            n211 = Power Of X(1:4.08, 2:2.0 ("x")) -> (0:w320:dbl)
            n212 = Power Of X(1:2.18, 2:4.0 ("x")) -> (0:w321:dbl)
            n213 = Subtract(x=w142, y=w181) -> (x-y=w189:dbl[])
            n214 = Reciprocal(x="t_dyz band") -> (1/x=w211:dbl)
            "dyz SDOS top \n(/eV/atom)" <- w211
            n215 = Multiply(x="t_dyz band", y=2.0) -> (x*y=w209:dbl)
            n216 = Subtract(x=w142, y="e_dyz band \n(vs. E_F)") -> (x-y=w207:dbl[])
            n217 = Divide(x=w321, y=w320) -> (x/y=w314:dbl)
            n218 = Divide(x=w207, y=w209) -> (x/y=w205:dbl[])
            n219 = Square(x=w205) -> (x^2=w204:dbl[])
            n220 = Subtract(x=1.0, y=w204) -> (x-y=w203:dbl[])
            n221 = Square Root(x=w203) -> (sqrt(x)=w202:dbl[])
            n222 = Multiply(x=w202, y=w211) -> (x*y=w201:dbl[])
            n223 = Add(x=w201, y=0.0) -> (x+y=w199:dbl[])
            n224 = Multiply(x="beta (per n)", y="mol backbone (# n)") -> (x*y=w331:dbl)
            n225 = for {
              tunnel: w199 -> [w433] mode=indexing
              tunnel: [w435] -> w187 mode=indexing
              n226 = Not A Number/Path/Refnum?(number/path/refnum=w433) -> (NaN/Path/Refnum?=w436:bool)
              n227 = Select(t=0.0, s=w436, f=w433) -> (s? t:f=w435:dbl)
            }
            n228 = Negate(x=w331) -> (-x=w386:dbl)
            n229 = Exponential(1:w386) -> (0:w330:dbl)
            n230 = Multiply(x=w187, y=w167) -> (x*y=w197:dbl[])
            n231 = call <vilib>:"Fast Hilbert Transform.vi"("X"=w197) -> ("Hilbert{X}"=w190:dbl[])  [unwired: 1 out]
            n232 = Subtract(x=w189, y=w190) -> (x-y=w191:dbl[])
            n233 = Multiply(x=w170, y=w169) -> (x*y=w123:dbl)
            n234 = Multiply(x=w119, y=w168) -> (x*y=w178:dbl)
            n235 = Multiply(x=w172, y=w171) -> (x*y=w124:dbl)
            n236 = Multiply(x=w122, y=w121) -> (x*y=w120:dbl)
            n237 = Bundle("Ramp Pattern"=w142, w189) -> (w186:cluster{"Ramp Pattern":dbl[], dbl[]})  [unwired: 1 in]
            n238 = Bundle("Ramp Pattern"=w142, w197) -> (w184:cluster{"Ramp Pattern":dbl[], dbl[]})  [unwired: 1 in]
            n239 = Absolute Value(x=w191) -> (abs(x)=w196:dbl[])
            n240 = Bundle("Ramp Pattern"=w142, "Hilbert{X}"=w190) -> (w185:T1)  [unwired: 1 in]
            n241 = for {
              tunnel: w196 -> [w432] mode=indexing
              tunnel: [w430] -> w192 mode=indexing if=w431
              tunnel: w142 -> [w430] mode=indexing
              n242 = Less Or Equal?(x=w432, y=0.01) -> (x <= y?=w431:bool)
            }
            n243 = Build Array(w186, w185, w184) -> (→"graphical sol_dyz band-mol":T2)
            n244 = Compound Arithmetic op=ADD(w124, w120, w123) -> (w179:dbl)
            n245 = Array Size(array=w192) -> (size(s)=w194:i32)
            n246 = Decrement(x=w194) -> (x-1=w195:i32)
            n247 = Index Array(array=w192, index #1=0 ("index"), index #2=w195) -> (element #2=w180:dbl)  [unwired: 1 out]
            "final ELA (eV), via \n(1) sp intercept\n(2) dz2 intercept\n(3) dyz intercept" <- w180
            "intercept on E\ndyz band-mol" <- w180
            n248 = Subtract(x=w142, y=w180) -> (x-y=w392:dbl[])
            n249 = Square(x=w392) -> (x^2=w326:dbl[])
            n250 = Threshold 1D Array(2:w180, 3:w142) -> (0:w188:dbl)  [unwired: 1 in]
            n251 = Subtract(x=w180, y=w181) -> (x-y=w174:dbl)
            "delta shift by d band \n(w.r.t. e_FMO coupled to s/p then dz2 )" <- w174
            n252 = Index Array(array=w187, index=w188) -> (element=w118:dbl)
            "unweighted dyz SDOS \n@intercept" <- w118
            n253 = Multiply(x=w118, y=w167) -> (x*y=w177:dbl)
            n254 = Compound Arithmetic op=ADD(w124, w120, w123, w178, w177) -> (w233:dbl)
            n255 = Square(x=w233) -> (x^2=w316:dbl)
            n256 = Divide(x=w316, y=4.0 ("x")) -> (x/y=w324:dbl)
            n257 = Add(x=w326, y=w324) -> (x+y=w325:dbl[])
            n258 = Compound Arithmetic op=ADD(w178, w177) -> (w176:dbl)
            n259 = Compound Arithmetic op=ADD(w119, w118) -> (w117:dbl)
            n260 = Divide(x=w233, y=w325) -> (x/y=w384:dbl[])
            n261 = Square(x=w384) -> (x^2=w315:dbl[])
            n262 = Multiply(x=w330, y=w315) -> (x*y=w327:dbl[])
            n263 = Multiply(x=w314, y=w327) -> (x*y=w236:dbl[])
            n264 = Array Max & Min(array=w236) -> (max value=w246:dbl, max index (indices)=w238:i32)  [unwired: 2 out]
            "peak value" <- w246
            n265 = Threshold 1D Array(2:0.0 ("threshold y"), 3:w142) -> (0:w389:dbl)  [unwired: 1 in]
            n266 = Index Array(array=w236, index=w389) -> (element=w232:dbl)
            "conductance G0 \n(on E_F, low bias)" <- w232
            n267 = Bundle("Ramp Pattern"=w142, w236) -> (→"transmission T(E)":cluster{"Ramp Pattern":dbl[], dbl[]})  [unwired: 1 in]
            n268 = Divide(x=w246, y=2.0) -> (x/y=w244:dbl)
            n269 = Threshold 1D Array(2:w244, 3:w236) -> (0:w240:dbl)  [unwired: 1 in]
            n270 = Compound Arithmetic op=ADD(w174, w175) -> (w173:dbl)
            n271 = Greater?(x=w232, y=1.0) -> (0:w280:bool)
            n272 = Index Array(array=w142, index=w238) -> (element=w237:dbl)
            n273 = Index Array(array=w142, index=w240) -> (element=w239:dbl)
            n274 = Absolute Value(x=w180) -> (abs(x)=w313:dbl)
            n275 = Subtract(x=w237, y=w239) -> (x-y=w243:dbl)
            n276 = Select(t=1.0 ("y"), s=w280, f=w232) -> (s? t:f=w231:dbl)
            n277 = Absolute Value(x=w243) -> (abs(x)=w242:dbl)
            n278 = Multiply(x=w242, y=2.0) -> (x*y=→"FWHM (eV)":dbl)
          }
          "e_FMO (y)" <- w110
        }
        "angle\narray\nfor sigma" <- w32
        n279 = Delete From Array(array=w7, index (col)=0 ("disabled index (col)")) -> ()  [unwired: 2 in, 2 out]
        n280 = Logarithm Base 10(1:w7) -> (0:w15:dbl[][])
        "log(G/G0) matrix" <- w15
        n281 = local read "e_FMO (y)"() -> (w4:dbl[])
        n282 = local read "angle\narray\nfor sigma"() -> (w5:dbl[])
        n283 = call-poly <vilib>:"Plot Helper.vi"("z matrix"=w15, "y vector"=w4, "x vector"=w5) -> ("3D Plot lvclass Array out"=→"log(G/G0)=f(angle, e_iso) for t(d-head)":refnum<class "3D Plot Datatype.lvclass">[])  [unwired: 3 in, 5 out]
        n284 = call-poly <vilib>:"Plot Helper.vi"("z matrix"=w13, "y vector"=w4, "x vector"=w5) -> ("3D Plot lvclass Array out"=→"Gamma(angle, e_iso) for t(d-head)_sum dz2 & dyz":refnum<class "3D Plot Datatype.lvclass">[])  [unwired: 3 in, 5 out]
        n285 = call-poly <vilib>:"Plot Helper.vi"("z matrix"=w3, "y vector"=w4, "x vector"=w5) -> ("3D Plot lvclass Array out"=→"SDOS(angle, e_iso) for t(d-head)_sum dz2 & dyz 2":refnum<class "3D Plot Datatype.lvclass">[])  [unwired: 3 in, 5 out]
        n286 = call-poly <vilib>:"Plot Helper.vi"("z matrix"=w14, "y vector"=w4, "x vector"=w5) -> ("3D Plot lvclass Array out"=→"Gamma(angle, e_iso) for t(sp-head)_sum s pz py":refnum<class "3D Plot Datatype.lvclass">[])  [unwired: 3 in, 5 out]
        n287 = call-poly <vilib>:"Plot Helper.vi"("z matrix"=w12, "y vector"=w4, "x vector"=w5) -> ("3D Plot lvclass Array out"=→"final ELA(angle, e_iso)  for t(d-head)":refnum<class "3D Plot Datatype.lvclass">[])  [unwired: 3 in, 5 out]
        n288 = call-poly <vilib>:"Plot Helper.vi"("z matrix"=w10, "y vector"=w4, "x vector"=w5) -> ("3D Plot lvclass Array out"=→"delta(angle, e_iso) for t(d-head)_sum dz2 & dyz":refnum<class "3D Plot Datatype.lvclass">[])  [unwired: 3 in, 5 out]
        n289 = call-poly <vilib>:"Plot Helper.vi"("z matrix"=w15, "y vector"=w4, "x vector"=w5) -> ("3D Plot lvclass Array out"=→"log(G/G0)=f(angle, e_iso) for t(sp-head)":refnum<class "3D Plot Datatype.lvclass">[])  [unwired: 3 in, 5 out]
        n290 = call-poly <vilib>:"Plot Helper.vi"("z matrix"=w11, "y vector"=w4, "x vector"=w5) -> ("3D Plot lvclass Array out"=→"delta(angle, e_iso) for t(sp-head)_only s":refnum<class "3D Plot Datatype.lvclass">[])  [unwired: 3 in, 5 out]
        n291 = call-poly <vilib>:"Plot Helper.vi"("z matrix"=w12, "y vector"=w4, "x vector"=w5) -> ("3D Plot lvclass Array out"=→"final ELA(angle, e_iso  for t(sp-head))":refnum<class "3D Plot Datatype.lvclass">[])  [unwired: 3 in, 5 out]
        n292 = case shown="True" "save heatmap \n(sp band)?" {
          tunnel: w15 -> [_ w89]
          tunnel: w20 -> [_ w82]
          tunnel: w19 -> [_ w81]
          tunnel: "_delta shift=f(t, e_iso)" ("string") -> [_ w80]
          tunnel: w16 -> [_ w79]
          tunnel: w14 -> [_ w78]
          tunnel: w12 -> [_ w77]
          tunnel: w11 -> [_ w76]
          tunnel: w5 -> [_ w71]
          frame False {
          }
          frame True {
            w69 = ".txt"
            w68 = "_t(sp band-anchor) " ("string")
            w74 = TRUE ("transpose? (no:F)")
            w75 = "%#.10f" ("format (%.3f)")
            n293 = Concatenate Strings("name (sp band)", w68, w69) -> (w67:string)
            n294 = Concatenate Strings("name (sp band)", w82, w68, w69) -> (w90:string)
            n295 = Concatenate Strings("name (sp band)", w81, w68, w69) -> (w88:string)
            n296 = Concatenate Strings("name (sp band)", w80, w68, w69) -> (w86:string)
            n297 = Concatenate Strings("name (sp band)", w79, w68, w69) -> (w84:string)
            n298 = Build Path(base path="saving path_heatmap (sp band)", name or relative path=w67) -> (appended path=w72:path)
            n299 = Build Path(base path="saving path_heatmap (sp band)", name or relative path=w90) -> (appended path=w73:path)
            n300 = Build Path(base path="saving path_heatmap (sp band)", name or relative path=w88) -> (appended path=w87:path)
            n301 = Build Path(base path="saving path_heatmap (sp band)", name or relative path=w86) -> (appended path=w85:path)
            n302 = Build Path(base path="saving path_heatmap (sp band)", name or relative path=w84) -> (appended path=w83:path)
            n303 = call-poly <vilib>:"Write Delimited Spreadsheet.vi"("file path (dialog if empty)"=w72, "format (%.3f)"=w75, "1D data"=w71, "transpose? (no:F)"=w74) -> ()  [unwired: 10 in, 2 out]
            n304 = call-poly <vilib>:"Write Delimited Spreadsheet.vi"("file path (dialog if empty)"=w73, "format (%.3f)"=w75, "2D data"=w89, "transpose? (no:F)"=w74) -> ()  [unwired: 10 in, 2 out]
            n305 = call-poly <vilib>:"Write Delimited Spreadsheet.vi"("file path (dialog if empty)"=w87, "format (%.3f)"=w75, "2D data"=w78, "transpose? (no:F)"=w74) -> ()  [unwired: 10 in, 2 out]
            n306 = call-poly <vilib>:"Write Delimited Spreadsheet.vi"("file path (dialog if empty)"=w85, "format (%.3f)"=w75, "2D data"=w76, "transpose? (no:F)"=w74) -> ()  [unwired: 10 in, 2 out]
            n307 = call-poly <vilib>:"Write Delimited Spreadsheet.vi"("file path (dialog if empty)"=w83, "format (%.3f)"=w75, "2D data"=w77, "transpose? (no:F)"=w74) -> ()  [unwired: 10 in, 2 out]
          }
        }
        n308 = case shown="True" "save heatmap \n(d band)?" {
          tunnel: w20 -> [_ w57]
          tunnel: w19 -> [_ w56]
          tunnel: "_delta shift=f(t, e_iso)" ("string") -> [_ w55]
          tunnel: w16 -> [_ w54]
          tunnel: w15 -> [_ w53]
          tunnel: w13 -> [_ w52]
          tunnel: w12 -> [_ w51]
          tunnel: w10 -> [_ w50]
          tunnel: w5 -> [_ w47]
          tunnel: "_SDOS=f(t, e_iso)" ("string") -> [_ w38]
          tunnel: w3 -> [_ w39]
          frame False {
          }
          frame True {
            w41 = "_t(d band-anchor) " ("string")
            w40 = ".txt"
            w44 = "%#.10f" ("format (%.3f)")
            w43 = TRUE ("transpose? (no:F)")
            n309 = Concatenate Strings("name (d band)", w41, w40) -> (w49:string)
            n310 = Concatenate Strings("name (d band)", w56, w41, w40) -> (w60:string)
            n311 = Concatenate Strings("name (d band)", w57, w41, w40) -> (w58:string)
            n312 = Concatenate Strings("name (d band)", w55, w41, w40) -> (w62:string)
            n313 = Concatenate Strings("name (d band)", w38, w41, w40) -> (w45:string)
            n314 = Concatenate Strings("name (d band)", w54, w41, w40) -> (w64:string)
            n315 = Build Path(base path="saving path_heatmap (d band)", name or relative path=w49) -> (appended path=w48:path)
            n316 = Build Path(base path="saving path_heatmap (d band)", name or relative path=w60) -> (appended path=w61:path)
            n317 = Build Path(base path="saving path_heatmap (d band)", name or relative path=w58) -> (appended path=w59:path)
            n318 = Build Path(base path="saving path_heatmap (d band)", name or relative path=w62) -> (appended path=w63:path)
            n319 = Build Path(base path="saving path_heatmap (d band)", name or relative path=w64) -> (appended path=w65:path)
            n320 = Build Path(base path="saving path_heatmap (d band)", name or relative path=w45) -> (appended path=w46:path)
            n321 = call-poly <vilib>:"Write Delimited Spreadsheet.vi"("file path (dialog if empty)"=w48, "format (%.3f)"=w44, "1D data"=w47, "transpose? (no:F)"=w43) -> ()  [unwired: 10 in, 2 out]
            n322 = call-poly <vilib>:"Write Delimited Spreadsheet.vi"("file path (dialog if empty)"=w61, "format (%.3f)"=w44, "2D data"=w52, "transpose? (no:F)"=w43) -> ()  [unwired: 10 in, 2 out]
            n323 = call-poly <vilib>:"Write Delimited Spreadsheet.vi"("file path (dialog if empty)"=w46, "format (%.3f)"=w44, "2D data"=w39, "transpose? (no:F)"=w43) -> ()  [unwired: 10 in, 2 out]
            n324 = call-poly <vilib>:"Write Delimited Spreadsheet.vi"("file path (dialog if empty)"=w59, "2D data"=w53, "transpose? (no:F)"=w43) -> ()  [unwired: 11 in, 2 out]
            n325 = call-poly <vilib>:"Write Delimited Spreadsheet.vi"("file path (dialog if empty)"=w63, "format (%.3f)"=w44, "2D data"=w50, "transpose? (no:F)"=w43) -> ()  [unwired: 10 in, 2 out]
            n326 = call-poly <vilib>:"Write Delimited Spreadsheet.vi"("file path (dialog if empty)"=w65, "format (%.3f)"=w44, "2D data"=w51, "transpose? (no:F)"=w43) -> ()  [unwired: 10 in, 2 out]
          }
        }
      }
      event Timeout {
        n327 = event-data() -> ()  [unwired: 1 in, 3 out]
      }
    }
  }
